vi "Enabled & Disabled.vi"() -> ()   [LabVIEW 2018]
panel:
  in  "Stop":bool
  in  "Run":bool
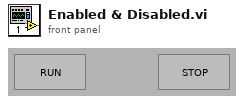
[diagram p1: front panel]
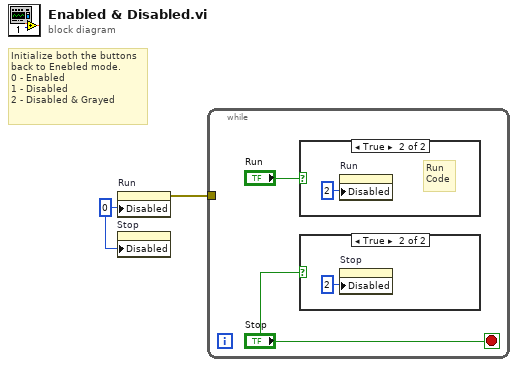
[diagram p0: block diagram]
diagram:
  w1 = u8 0 ("Disabled")
  # "Initialize both the buttons\nback to Enebled mode.\n0 - Enabled\n1 - Disabled\n2 - Disabled & Grayed"
  n1 = property on="Run" class="Bool"("Disabled"=w1) -> (error out=w2:errorcluster)  [unwired: 2 in, 1 out]
  n2 = property on="Stop" class="Bool"("Disabled"=w1) -> ()  [unwired: 2 in, 2 out]
  n3 = while {
    tunnel: w2 -> [_]
    stop <- "Stop" stop-if-true
    n4 = case shown="True" "Run" {
      frame False {
      }
      frame True {
        # "Run\nCode"
        n5 = property on="Run" class="Bool"("Disabled"=u8 2) -> ()  [unwired: 2 in, 2 out]
      }
    }
    n6 = case shown="True" "Stop" {
      frame False {
      }
      frame True {
        n7 = property on="Stop" class="Bool"("Disabled"=u8 2) -> ()  [unwired: 2 in, 2 out]
      }
    }
  }
